vi "serpenbot_DDPG_control_parallel_old_camera_1.vi"() -> ()   [LabVIEW 2020]
uses:
  <vilib>/Analysis/Matrix/Datatypes/RealMatrix.ctl
  <vilib>/Analysis/Matrix/NI_Matrix.lvlib
  <vilib>/Analysis/NI_AALPro.lvlib
  <vilib>/Analysis/_algsub.llb/Real PseudoInverse Matrix.vi
  <vilib>/Analysis/NI_AALBase.lvlib
  <vilib>/Analysis/baseanly.llb/Real A x B.vi
  <vilib>/Analysis/Matrix/Numeric/Subtract/Subtract - RM,RM.vi
panel:
  out "camera_value 2":T1
  out "appended array 3":T1
  out "error out Y":errorcluster
  out "error out X":errorcluster
  in  "goal y":dbl
  in  "goal x":dbl
  in  "k":T1
  out "control_loop_time":u32
  in  "stop":bool
  in  "Logging":bool caption="Enable"
  out "current x":dbl
  out "current y":dbl
  out "laser control value":dbl[](array[numeric])
  in  "Diode Current\nSetting":dbl=3.0
  in  "Laser Repetition\nFrequency":i32=50000
  in  "VISA resource name":refnum<visa-resource-name>="COM14"
  in  "baud rate (9600)":u32=9600
  out "error out":errorcluster
  out "Identification system 1":string
  out "Conn. axes system 1":string[](array[string])
  out "Identification system 2":string
  out "Conn. axes system  2":string[](array[string])
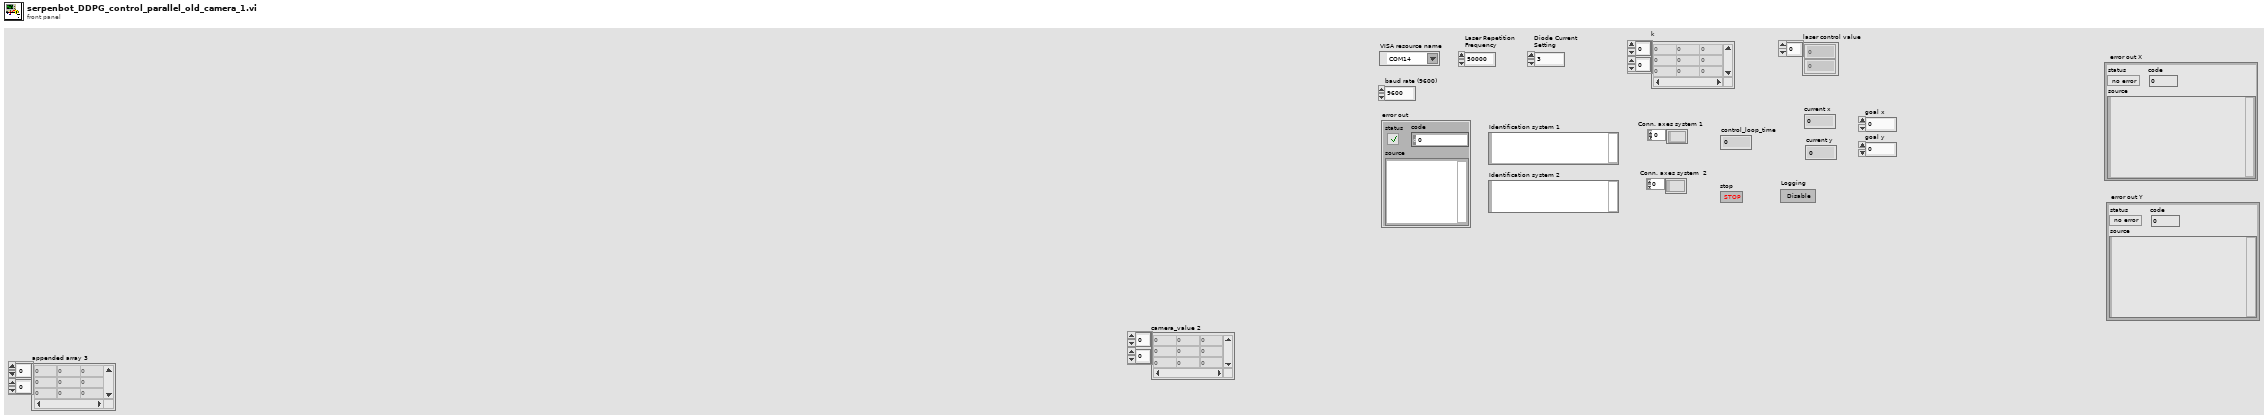
[diagram p1: front panel]
types:
  T1 = typedef "NI_Matrix.lvlib/RealMatrix.ctl" = dbl[][]
  T2 = cluster{"RS232 settings":cluster{"Portnumber":i32, "Baudrate":u16}, "USB settings":cluster{"S/N":string, "USB Search?":bool}, "TCP/IP settings":cluster{"Host address/name":string, "Port":i32, "Board":i32, "TCP/IP Search?":bool}}
  T3 = cluster{"Check FRF?":bool, "Referencing mode":enum16{"FRF (-> FNL)", "FRF", "FNL", "FPL", "RON OFF"}[]}
  T4 = cluster{"Force?":bool, "Dialog?":bool, "Stages":string[]}
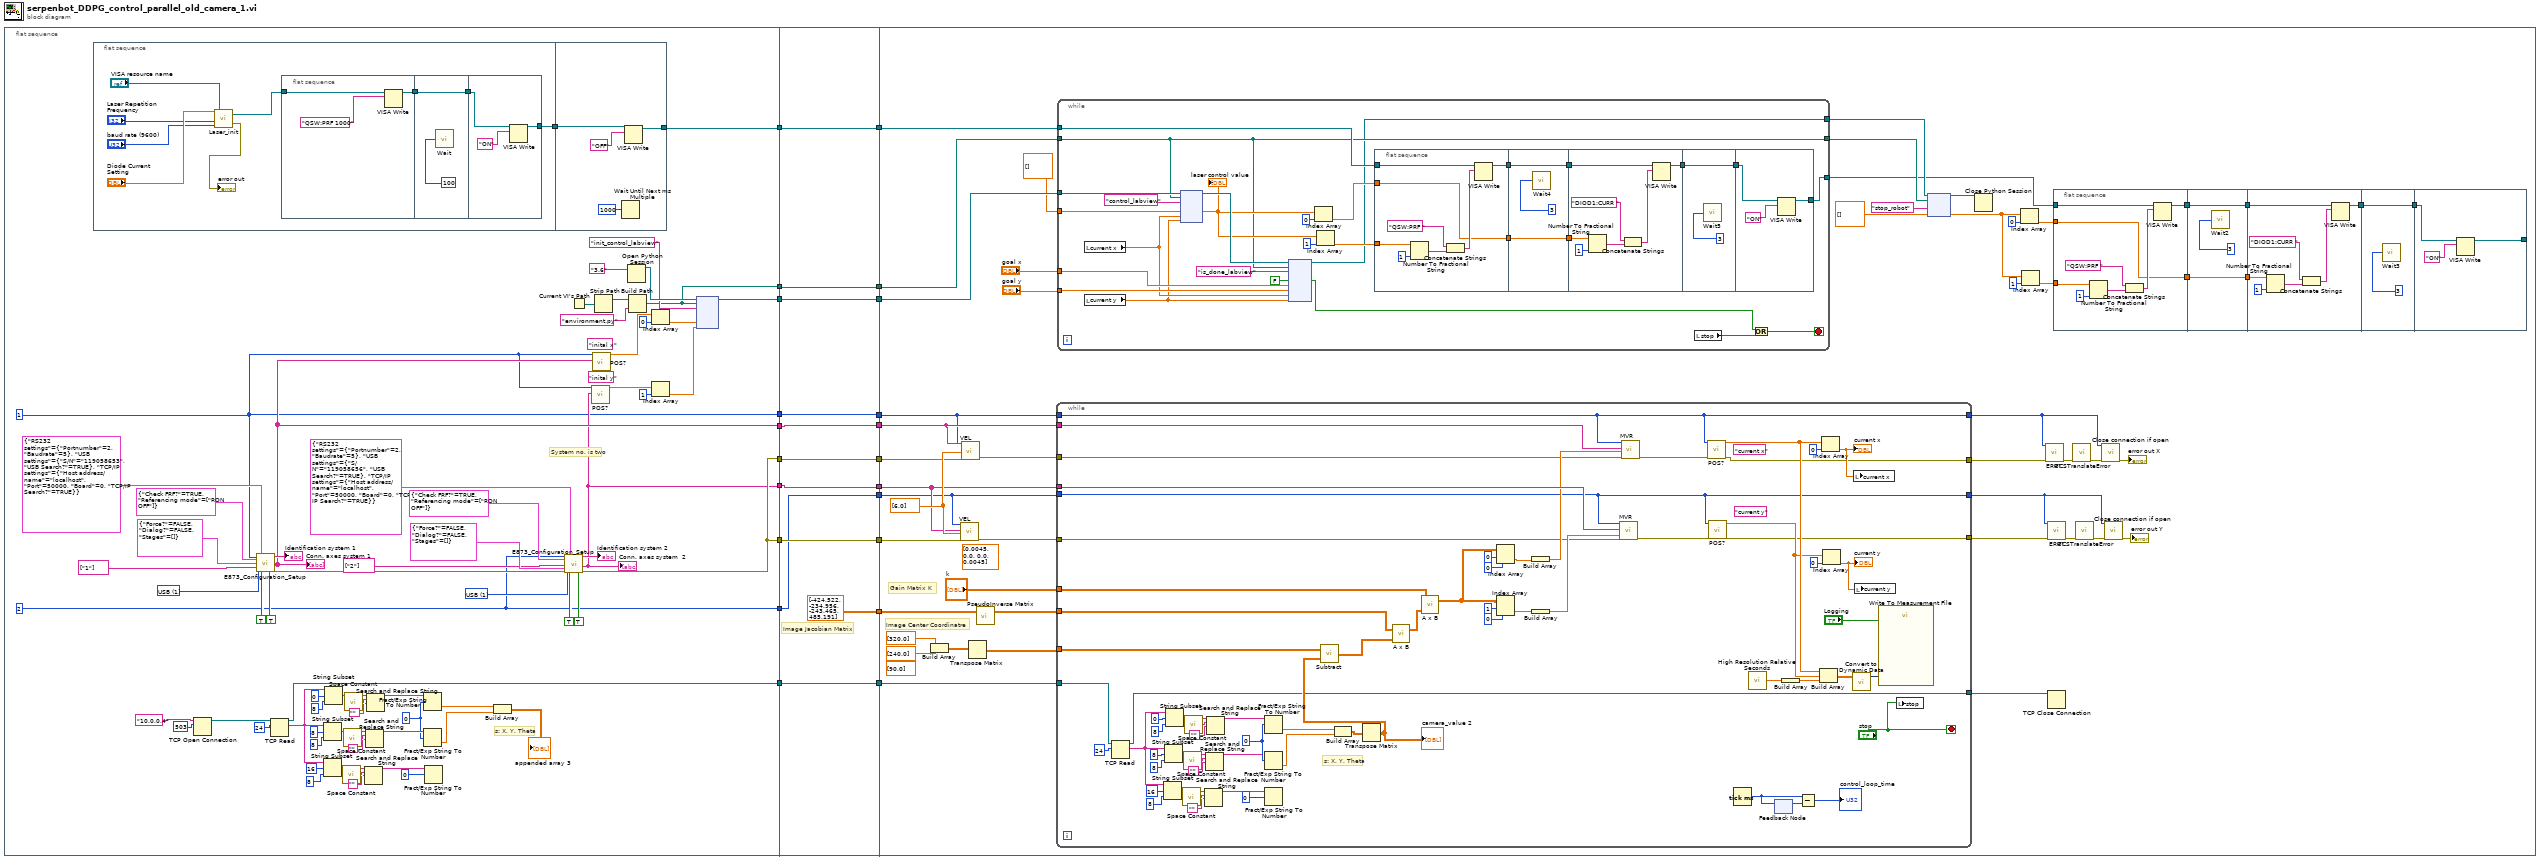
[diagram p0: block diagram]
diagram:
  n1 = flat-sequence {
    tunnel: [w87] -> w21
    tunnel: [w57] -> w20
    tunnel: [w59] -> w19
    tunnel: [w68] -> w18
    tunnel: [w58] -> w17
    tunnel: [w69] -> w16
    tunnel: [w68] -> w15
    tunnel: [w61] -> w14
    tunnel: [w60] -> w13
    tunnel: [w22] -> w1
    tunnel: w21 -> [w120]
    tunnel: [w120] -> w12
    tunnel: w20 -> [w119]
    tunnel: w19 -> [w118]
    tunnel: w18 -> [w117]
    tunnel: w17 -> [w116]
    tunnel: w16 -> [w114]
    tunnel: [w119] -> w11
    tunnel: [w118] -> w10
    tunnel: [w117] -> w9
    tunnel: [w116] -> w8
    tunnel: w15 -> [w115]
    tunnel: [w115] -> w7
    tunnel: [w114] -> w6
    tunnel: [T1 [[-424.522, -234.956], [-243.465, 485.191]] ("J_init 2")] -> w5
    tunnel: w14 -> [w112]
    tunnel: w13 -> [w111]
    tunnel: [w112] -> w4
    tunnel: [w111] -> w3
    tunnel: [w110] -> w2
    tunnel: w1 -> [w110]
    tunnel: w12 -> [w139]
    tunnel: w11 -> [w157]
    tunnel: w10 -> [w164]
    tunnel: w9 -> [w167]
    tunnel: w8 -> [w162]
    tunnel: w7 -> [w166]
    tunnel: w6 -> [w156]
    tunnel: w5 -> [w165]
    tunnel: w4 -> [w141]
    tunnel: w3 -> [w140]
    tunnel: w2 -> [w122]
    frame #0 {
      w36 = 0
      (unwired) "inital y"
      (unwired) "inital x"
      w72 = u16 1 items=["RS232", "USB", "TCP/IP"] ("Interface")
      w75 = u16 1 items=["RS232", "USB", "TCP/IP"] ("Interface")
      w69 = 2 ("System no.")
      w57 = 1 ("System no.")
      # "s: X, Y, Theta"
      # "System no. is two"
      n2 = flat-sequence {
        tunnel: [w89] -> w88
        tunnel: w88 -> [w107]
        tunnel: [w106] -> w87
        frame #0 {
          n3 = call "Laser_init.vi"("baud rate (9600)"="baud rate (9600)", "Laser Repetition\nFrequency"="Laser Repetition\nFrequency", "VISA resource name"="VISA resource name", "Diode Current\nSetting"="Diode Current\nSetting") -> ("error out"=→"error out":errorcluster, "VISA Refnum out"=w90:refnum<visa-resource-name>)
          n4 = flat-sequence {
            tunnel: w90 -> [w100]
            tunnel: [w99] -> w97
            tunnel: w97 -> [w102]
            tunnel: [w102] -> w96
            tunnel: w96 -> [w103]
            tunnel: [w104] -> w89
            frame #0 {
              n5 = VISA Write(VISA resource name=w100, write buffer="QSW:PRF 1000" ("string")) -> (VISA resource name out=w99:refnum<visa-resource-name>)  [unwired: 1 in, 2 out]
            }
            frame #1 {
              n6 = call "Wait"("Count(mSec)"=u32 100) -> ()  [unwired: 1 out]
            }
            frame #2 {
              n7 = VISA Write(VISA resource name=w103, write buffer="ON") -> (VISA resource name out=w104:refnum<visa-resource-name>)  [unwired: 1 in, 2 out]
            }
          }
        }
        frame #1 {
          n8 = Wait Until Next ms Multiple(millisecond multiple=u32 1000) -> ()  [unwired: 1 out]
          n9 = VISA Write(VISA resource name=w107, write buffer="OFF") -> (VISA resource name out=w106:refnum<visa-resource-name>)  [unwired: 1 in, 2 out]
        }
      }
      n10 = TCP Open Connection(address="10.0.0.4", remote port or service name=u16 503) -> (connection ID=w46:refnum<k5>)  [unwired: 3 in, 1 out]
      n11 = call "E873_Configuration_Setup.vi"("System no."=w57, "Referencing"=T3 {"Check FRF?"=TRUE, "Referencing mode"=[enum."RON OFF"]}, "Interface"=w75, "All axes?"=TRUE, "Axes to move"=string[] ["1"], "Interface settings"=T2 {"RS232 settings"={"Portnumber"=2, "Baudrate"=5}, "USB settings"={"S/N"="119058653", "USB Search?"=TRUE}, "TCP/IP settings"={"Host address/name"="localhost", "Port"=50000, "Board"=0, "TCP/IP Search?"=TRUE}}, "Stage selection"=T4 {"Force?"=FALSE, "Dialog?"=FALSE, "Stages"=[]}, "Switch servo on?"=TRUE ("Use dialog to define\nconnected stages?")) -> ("Identification"=→"Identification system 1":string, "Conn. \nAxes"=w59:string[], "error out"=w84:errorcluster)  [unwired: 4 in, 5 out]
      "Conn. axes system 1" <- w59
      n12 = TCP Read(connection ID=w46, bytes to read=24) -> (connection ID out=w22:refnum<k5>, data out=w45:string)  [unwired: 3 in, 1 out]
      n13 = String Subset(string=w45, offset (0)=16, length (rest)=8 ("length (rest)")) -> (substring=w43:string)
      n14 = String Subset(string=w45, offset (0)=8, length (rest)=8 ("length (rest)")) -> (substring=w44:string)
      n15 = String Subset(string=w45, offset (0)=0, length (rest)=8 ("length (rest)")) -> (substring=w42:string)
      n16 = call <vilib>:"Space Constant.vi"() -> ("String"=w41:string)
      n17 = call <vilib>:"Space Constant.vi"() -> ("String"=w40:string)
      n18 = call <vilib>:"Space Constant.vi"() -> ("String"=w39:string)
      n19 = Search and Replace String(input string=w43, search string=w41, replace string="") -> (result string=w47:string)  [unwired: 5 in, 3 out]
      n20 = Search and Replace String(input string=w44, search string=w40, replace string="") -> (result string=w48:string)  [unwired: 5 in, 3 out]
      n21 = Search and Replace String(input string=w42, search string=w39, replace string="") -> (result string=w49:string)  [unwired: 5 in, 3 out]
      n22 = Fract/Exp String To Number(string=w49, offset=w36) -> (number=w37:dbl)  [unwired: 2 in, 1 out]
      n23 = Fract/Exp String To Number(string=w48, offset=w36) -> (number=w38:dbl)  [unwired: 2 in, 1 out]
      n24 = Fract/Exp String To Number(string=w47, offset=0) -> ()  [unwired: 2 in, 2 out]
      n25 = Build Array(w37, w38) -> (→"appended array 3":T1)
      n26 = call "E873_Configuration_Setup.vi"("System no."=w69, "Referencing"=T3 {"Check FRF?"=TRUE, "Referencing mode"=[enum."RON OFF"]}, "Interface"=w72, "All axes?"=TRUE, "Axes to move"=string[] ["2"], "error in"=w84, "Interface settings"=T2 {"RS232 settings"={"Portnumber"=2, "Baudrate"=5}, "USB settings"={"S/N"="119058656", "USB Search?"=TRUE}, "TCP/IP settings"={"Host address/name"="localhost", "Port"=50000, "Board"=0, "TCP/IP Search?"=TRUE}}, "Stage selection"=T4 {"Force?"=FALSE, "Dialog?"=FALSE, "Stages"=[]}, "Switch servo on?"=TRUE ("Use dialog to define\nconnected stages?")) -> ("Identification"=→"Identification system 2":string, "Conn. \nAxes"=w58:string[], "error out"=w68:errorcluster)  [unwired: 3 in, 5 out]
      "Conn. axes system  2" <- w58
      n27 = Current VI's Path() -> (path=w67:path)
      n28 = call "POS?.vi"("System no."=w57, "Axes to query"=w58) -> ("Position"=w52:dbl[])  [unwired: 3 in, 14 out]
      n29 = call "POS?.vi"("System no."=w57, "Axes to query"=w59) -> ("Position"=w54:dbl[])  [unwired: 3 in, 14 out]
      n30 = Strip Path(path=w67) -> (stripped path=w66:path)  [unwired: 1 out]
      n31 = Open Python Session(python version="3.6" ("Python version")) -> (session out=w63:refnum<k35>)  [unwired: 2 in, 1 out]
      n32 = Build Path(base path=w66, name or relative path="environment.py") -> (appended path=w61:path)
      n33 = Index Array(array=w54, index=0) -> (element=w55:dbl)
      n34 = Index Array(array=w52, index=1) -> (element=w51:dbl)
      n35 = node(w63, w61, "init_control_labview" ("function name"), w55, w51) -> (w60:refnum<k35>)  [unwired: 5 in, 3 out]
    }
    frame #1 {
      # "Image Jacobian Matrix"
    }
    frame #2 {
      w168 = dbl[] [6.0] ("Velocity values")
      (unwired) T1 [[0.0045, 0.0], [0.0, 0.0045]] ("J_init 2")
      (unwired) dbl[] [90.0] ("element")
      # "Gain Matrix K"
      # "Image Center Coordinatre"
      n36 = Build Array(dbl[] [320.0] ("element"), dbl[] [240.0] ("element")) -> (w169:T1)
      n37 = call "VEL.vi"("System no."=w156, "Axes to set"=w162, "Velocity values"=w168, "error in"=w166) -> ("error out"=w161:errorcluster)  [unwired: 2 in, 13 out]
      n38 = call "VEL.vi"("System no."=w157, "Axes to set"=w164, "Velocity values"=w168, "error in"=w167) -> ("error out"=w163:errorcluster)  [unwired: 2 in, 13 out]
      n39 = Transpose Matrix(1:w169) -> (0:w158:T1)
      n40 = call-poly <vilib>:"PseudoInverse Matrix.vi"("Input Matrix"=w165) -> ("PseudoInverse Matrix"=w159:T1)  [unwired: 1 in, 1 out]
      n41 = while {
        tunnel: w161 -> [w271]
        tunnel: w156 -> [w252]
        tunnel: w162 -> [w289]
        tunnel: w163 -> [w272]
        tunnel: w164 -> [w288]
        tunnel: w157 -> [w254]
        tunnel: w159 -> [w277]
        tunnel: "k" -> [w276]
        tunnel: w158 -> [w275]
        tunnel: [w254] -> w125
        tunnel: [w253] -> w126
        tunnel: [w252] -> w124
        tunnel: [w251] -> w123
        tunnel: w122 -> [w224]
        tunnel: [w223] -> w121
        stop <- "stop" stop-if-true
        w250 = 0
        (unwired) "current y"
        (unwired) "current x"
        # "s: X, Y, Theta"
        n42 = TCP Read(connection ID=w224, bytes to read=24) -> (connection ID out=w223:refnum<k5>, data out=w231:string)  [unwired: 3 in, 1 out]
        n43 = String Subset(string=w231, offset (0)=16, length (rest)=8 ("length (rest)")) -> (substring=w233:string)
        n44 = String Subset(string=w231, offset (0)=8, length (rest)=8 ("length (rest)")) -> (substring=w232:string)
        n45 = String Subset(string=w231, offset (0)=0, length (rest)=8 ("length (rest)")) -> (substring=w238:string)
        n46 = call <vilib>:"Space Constant.vi"() -> ("String"=w241:string)
        n47 = call <vilib>:"Space Constant.vi"() -> ("String"=w243:string)
        n48 = call <vilib>:"Space Constant.vi"() -> ("String"=w245:string)
        n49 = Search and Replace String(input string=w233, search string=w241, replace string="") -> (result string=w229:string)  [unwired: 5 in, 3 out]
        n50 = Search and Replace String(input string=w232, search string=w243, replace string="") -> (result string=w228:string)  [unwired: 5 in, 3 out]
        n51 = Search and Replace String(input string=w238, search string=w245, replace string="") -> (result string=w227:string)  [unwired: 5 in, 3 out]
        n52 = Fract/Exp String To Number(string=w227, offset=w250) -> (number=w249:dbl)  [unwired: 2 in, 1 out]
        n53 = Fract/Exp String To Number(string=w228, offset=w250) -> (number=w248:dbl)  [unwired: 2 in, 1 out]
        n54 = Fract/Exp String To Number(string=w229, offset=0) -> ()  [unwired: 2 in, 2 out]
        n55 = Build Array(w249, w248) -> (w226:T1)
        n56 = Transpose Matrix(1:w226) -> (0:w225:T1)
        "camera_value 2" <- w225
        n57 = call-poly <vilib>:"Subtract.vi"("Real Matrix B"=w225, "Real Matrix A"=w275) -> ("A - B"=w283:T1)
        n58 = call-poly <vilib>:"A x B.vi"("B"=w283, "A"=w277) -> ("A x B"=w281:T1)  [unwired: 1 out]
        n59 = call-poly <vilib>:"A x B.vi"("B"=w281, "A"=w276) -> ("A x B"=w282:T1)  [unwired: 1 out]
        n60 = Index Array(array=w282, index (row)=0, index (col)=0) -> (element=w274:dbl)
        n61 = Index Array(array=w282, index (row)=1, index (col)=0) -> (element=w273:dbl)
        n62 = Build Array(w274) -> (w280:dbl[])
        n63 = Build Array(w273) -> (w279:dbl[])
        n64 = call "MVR.vi"("System no."=w252, "Axes to move"=w289, "Position values"=w279, "error in"=w271) -> ("error out"=w263:errorcluster)  [unwired: 1 in, 14 out]
        n65 = call "MVR.vi"("System no."=w254, "Axes to move"=w288, "Position values"=w280, "error in"=w272) -> ("error out"=w264:errorcluster)  [unwired: 1 in, 14 out]
        n66 = call "POS?.vi"("System no."=w254, "error in"=w264) -> ("Position"=w261:dbl[], "error out"=w253:errorcluster)  [unwired: 3 in, 13 out]
        n67 = call "POS?.vi"("System no."=w252, "error in"=w263) -> ("Position"=w259:dbl[], "error out"=w251:errorcluster)  [unwired: 3 in, 13 out]
        n68 = Tick Count (ms)() -> (millisecond timer value=w262:u32)
        n69 = call <vilib>:"High Resolution Relative Seconds.vi"() -> ("relative seconds"=w266:dbl)
        n70 = feedback #1() -> (w278:u32)  [unwired: 1 in]
        n71 = feedback-in #1(w262) -> ()
        n72 = Build Array(w266) -> (w265:dbl[])
        n73 = Subtract(x=w262, y=w278) -> (x-y=→"control_loop_time":u32)
        n74 = Build Array(w261, w259, w265) -> (w268:dbl[][])
        n75 = Index Array(array=w261, index=0) -> (element=w257:dbl)
        "current x" <- w257
        n76 = Index Array(array=w259, index=0) -> (element=w256:dbl)
        "current y" <- w256
        n77 = call "Convert to Dynamic Data"("2D Array"=w268) -> ("Dynamic Data Type"=w267:dynamicdata)  [unwired: 3 in]
        n78 = local write "current x"(w257) -> ()
        n79 = local write "current y"(w256) -> ()
        n80 = call "Write To Measurement File"("Signals"=w267, "Enable"="Logging") -> ()  [unwired: 15 in, 3 out]
        n81 = local write "stop"("stop") -> ()
      }
      n82 = while {
        tunnel: dbl[] [] -> [w184]
        tunnel: "goal x" -> [w183]
        tunnel: "goal y" -> [w182]
        tunnel: w141 -> [w179]
        tunnel: w140 -> [w181]
        tunnel: w139 -> [w180]
        tunnel: [w179] -> w138
        tunnel: [w178] -> w137
        tunnel: [w175] -> w136
        stop <- w176 stop-if-true
        n83 = local read "current x"() -> (w174:dbl)
        n84 = local read "current y"() -> (w173:dbl)
        n85 = node(w181, w179, "control_labview" ("function name"), w184, w174, w173) -> (w192:refnum<k35>, w186:dbl[])  [unwired: 3 in, 3 out]
        "laser control value" <- w186
        n86 = node(w192, w179, "is_done_labview" ("function name"), FALSE, w183, w182, w174, w173) -> (w178:refnum<k35>, w172:bool)  [unwired: 5 in, 3 out]
        n87 = Index Array(array=w186, index=0) -> (element=w189:dbl)
        n88 = Index Array(array=w186, index=1) -> (element=w185:dbl)
        n89 = flat-sequence {
          tunnel: w180 -> [w203]
          tunnel: [w202] -> w199
          tunnel: w185 -> [w201]
          tunnel: w189 -> [w200]
          tunnel: [w200] -> w198
          tunnel: [w210] -> w197
          tunnel: [w208] -> w196
          tunnel: w199 -> [w210]
          tunnel: w198 -> [w208]
          tunnel: [w217] -> w195
          tunnel: w197 -> [w215]
          tunnel: w196 -> [w212]
          tunnel: w195 -> [w219]
          tunnel: [w219] -> w194
          tunnel: w194 -> [w221]
          tunnel: [w220] -> w175
          frame #0 {
            n90 = Number To Fractional String(number=w201, precision (6)=i16 1) -> (F-format string=w206:string)  [unwired: 2 in]
            n91 = Concatenate Strings("QSW:PRF " ("string"), w206) -> (w207:string)
            n92 = VISA Write(VISA resource name=w203, write buffer=w207) -> (VISA resource name out=w202:refnum<visa-resource-name>)  [unwired: 1 in, 2 out]
          }
          frame #1 {
            n93 = call "Wait4"("Count(mSec)"=u32 3) -> ()  [unwired: 1 out]
          }
          frame #2 {
            n94 = Number To Fractional String(number=w212, precision (6)=i16 1) -> (F-format string=w213:string)  [unwired: 2 in]
            n95 = Concatenate Strings("DIOD1:CURR " ("string"), w213) -> (w216:string)
            n96 = VISA Write(VISA resource name=w215, write buffer=w216) -> (VISA resource name out=w217:refnum<visa-resource-name>)  [unwired: 1 in, 2 out]
          }
          frame #3 {
            n97 = call "Wait5"("Count(mSec)"=u32 3) -> ()  [unwired: 1 out]
          }
          frame #4 {
            n98 = VISA Write(VISA resource name=w221, write buffer="ON") -> (VISA resource name out=w220:refnum<visa-resource-name>)  [unwired: 1 in, 2 out]
          }
        }
        n99 = local read "stop"() -> (w177:bool)
        n100 = Or(x=w172, y=w177) -> (x .or. y?=w176:bool)
      }
      n101 = node(w137, w138, "stop_robot" ("function name"), dbl[] []) -> (w147:refnum<k35>, w142:dbl[])  [unwired: 1 in, 3 out]
      n102 = Close Python Session(session in=w147) -> ()  [unwired: 1 in, 1 out]
      n103 = Index Array(array=w142, index=0) -> (element=w144:dbl)
      n104 = Index Array(array=w142, index=1) -> (element=w143:dbl)
      n105 = call "ERR?.vi"("System no."=w125, "error in"=w126) -> ("error out"=w130:errorcluster)  [unwired: 17 out]
      n106 = call "ERR?.vi"("System no."=w124, "error in"=w123) -> ("error out"=w127:errorcluster)  [unwired: 17 out]
      n107 = TCP Close Connection(connection ID=w121) -> ()  [unwired: 2 in, 2 out]
      n108 = flat-sequence {
        tunnel: w136 -> [w293]
        tunnel: [w292] -> w155
        tunnel: w143 -> [w291]
        tunnel: w144 -> [w290]
        tunnel: [w290] -> w154
        tunnel: [w300] -> w153
        tunnel: [w298] -> w152
        tunnel: w155 -> [w300]
        tunnel: w154 -> [w298]
        tunnel: [w307] -> w151
        tunnel: w153 -> [w305]
        tunnel: w152 -> [w302]
        tunnel: w151 -> [w309]
        tunnel: [w309] -> w150
        tunnel: w150 -> [w311]
        tunnel: [w310] -> _
        frame #0 {
          n109 = Number To Fractional String(number=w291, precision (6)=i16 1) -> (F-format string=w296:string)  [unwired: 2 in]
          n110 = Concatenate Strings("QSW:PRF " ("string"), w296) -> (w297:string)
          n111 = VISA Write(VISA resource name=w293, write buffer=w297) -> (VISA resource name out=w292:refnum<visa-resource-name>)  [unwired: 1 in, 2 out]
        }
        frame #1 {
          n112 = call "Wait2"("Count(mSec)"=u32 3) -> ()  [unwired: 1 out]
        }
        frame #2 {
          n113 = Number To Fractional String(number=w302, precision (6)=i16 1) -> (F-format string=w303:string)  [unwired: 2 in]
          n114 = Concatenate Strings("DIOD1:CURR " ("string"), w303) -> (w306:string)
          n115 = VISA Write(VISA resource name=w305, write buffer=w306) -> (VISA resource name out=w307:refnum<visa-resource-name>)  [unwired: 1 in, 2 out]
        }
        frame #3 {
          n116 = call "Wait3"("Count(mSec)"=u32 3) -> ()  [unwired: 1 out]
        }
        frame #4 {
          n117 = VISA Write(VISA resource name=w311, write buffer="ON") -> (VISA resource name out=w310:refnum<visa-resource-name>)  [unwired: 1 in, 2 out]
        }
      }
      n118 = call "GCSTranslateError.vi"("error in"=w130) -> ("error out"=w131:errorcluster)  [unwired: 18 out]
      n119 = call "GCSTranslateError.vi"("error in"=w127) -> ("error out"=w128:errorcluster)  [unwired: 18 out]
      n120 = call "Close connection if open.vi"("System no."=w125, "error in"=w131) -> ("error out"=→"error out X":errorcluster)  [unwired: 1 in, 16 out]
      n121 = call "Close connection if open.vi"("System no."=w124, "error in"=w128) -> ("error out"=→"error out Y":errorcluster)  [unwired: 1 in, 16 out]
    }
  }
